vi "40 Nested Case Structures.vi"() -> ()   [LabVIEW 2018]
panel:
  in  "Switch 0":bool
  in  "Switch 1":bool
  in  "stop":bool
  out "C":dbl
  in  "B":dbl
  in  "A":dbl
  # "Divide"
  # "Multiply"
  # "Subtract"
  # "Add"
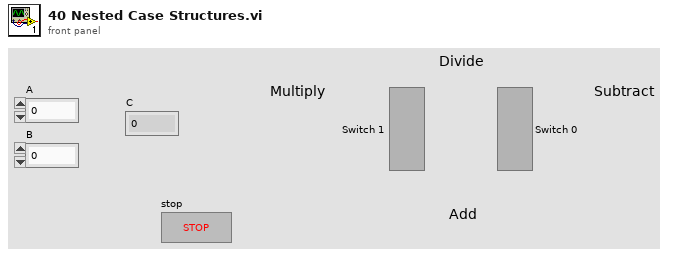
[diagram p1: front panel]
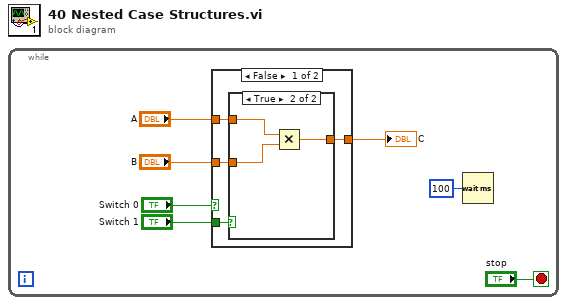
[diagram p0: block diagram]
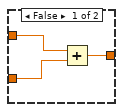
[diagram p2: hidden frame]
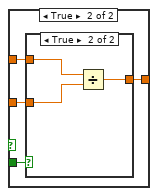
[diagram p3: hidden frame]
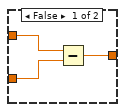
[diagram p4: hidden frame]
diagram:
  n1 = while {
    stop <- "stop" stop-if-true
    n2 = case shown="False" "Switch 0" {
      tunnel: "A" -> [w11 w21]
      tunnel: "B" -> [w10 w20]
      tunnel: [w9 w19] -> w5
      tunnel: "Switch 1" -> [w8 w18]
      frame False {
        n3 = case shown="True" w8 {
          tunnel: w11 -> [w14 w16]
          tunnel: w10 -> [w13 w15]
          tunnel: [w12 w17] -> w9
          frame False {
            n4 = Add(x=w14, y=w13) -> (x+y=w12:dbl)
          }
          frame True {
            n5 = Multiply(x=w16, y=w15) -> (x*y=w17:dbl)
          }
        }
      }
      frame True {
        n6 = case shown="True" w18 {
          tunnel: w21 -> [w24 w27]
          tunnel: w20 -> [w23 w26]
          tunnel: [w22 w25] -> w19
          frame False {
            n7 = Subtract(x=w24, y=w23) -> (x-y=w22:dbl)
          }
          frame True {
            n8 = Divide(x=w27, y=w26) -> (x/y=w25:dbl)
          }
        }
      }
    }
    "C" <- w5
    n9 = Wait (ms)(milliseconds to wait=u32 100) -> ()  [unwired: 1 out]
  }
